vi "Execute.vi"(8 "error in (no error)":errorcluster, 10 "Notify Plugins of Menu Up in":refnum<class "Notify Plugins of Menu Up.lvclass">, 11 "Plugin Handler Shifter Data Definition":T1) -> (0 "error out":errorcluster, 1 "Stop?":bool, 2 "Plugin Generic Command out":refnum<class "Plugin Handler Command.lvclass">, 3 "Plugin Handler Shifter Data Out":T1)   [LabVIEW 2011, in "Notify Plugins of Menu Up.lvclass"]
uses:
  Notify Plugins of Menu Up.lvclass
  Plugin Handler Command.lvclass
  Plugin Strict Type Definitions/Plugin Handler Shifter Data Definition.ctl
  Parent Plugin Definition/Plugin Template/Generic Plugin.lvclass
  Plugin Strict Type Definitions/Plugin Configuration Information.ctl
  User Interface/UI Command Manager/UI Command Manager.lvclass
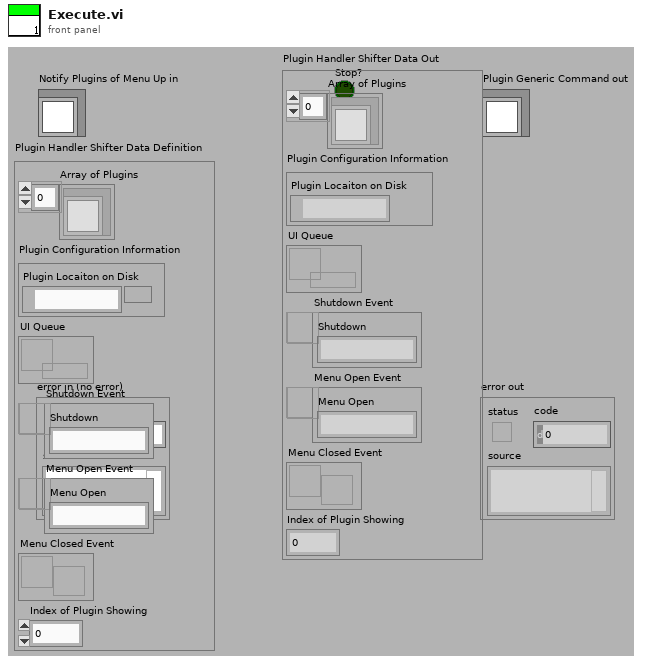
[diagram p1: front panel]
types:
  T1 = typedef "Plugin Handler Shifter Data Definition.ctl" = cluster{"Array of Plugins":refnum<class "Generic Plugin.lvclass">[], "Plugin Configuration Information":T2, "UI Queue":refnum<queue>, "Shutdown Event":refnum<user-event>, "Menu Open Event":refnum<user-event>, "Menu Closed Event":refnum<user-event>, "Index of Plugin Showing":i32}
  T2 = typedef "Plugin Configuration Information.ctl" = cluster{"Plugin Locaiton on Disk":path}
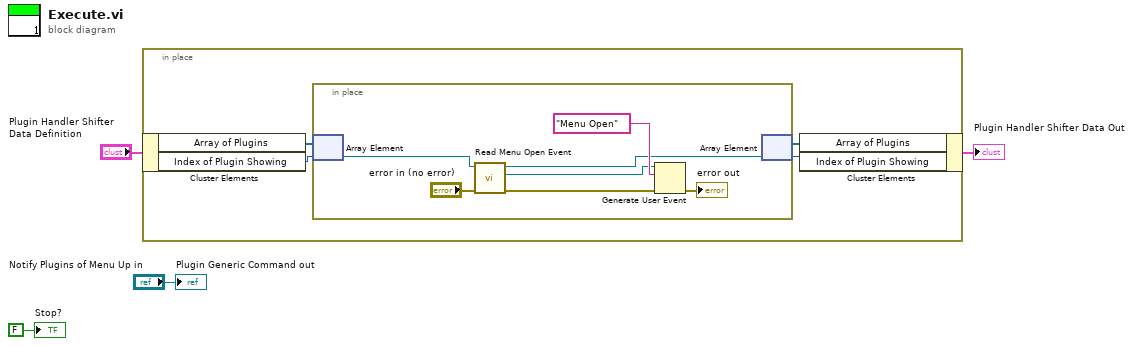
[diagram p0: block diagram]
diagram:
  n1 = in-place {
    n2 = in-place-cluster #1("Plugin Handler Shifter Data Definition") -> ("Array of Plugins"=w8:refnum<class "Generic Plugin.lvclass">[], "Index of Plugin Showing"=w7:i32)
    n3 = in-place {
      n4 = in-place-array #2(w8, w7) -> (w13:refnum<class "Generic Plugin.lvclass">)
      n5 = call "Read Menu Open Event.vi"("error in (no error)"="error in (no error)", "Generic Plugin in"=w13) -> ("error out"=w14:errorcluster, "Menu Open Event"=w12:refnum<user-event>, "Generic Plugin out"=w11:refnum<class "Generic Plugin.lvclass">)  [unwired: 7 in]
      n6 = Generate User Event(user event=w12, event data cluster="Menu Open" ("event data"), error in=w14) -> (error out=→"error out":errorcluster)  [unwired: 1 out]
      n7 = in-place-array #2(w11) -> (w6:refnum<class "Generic Plugin.lvclass">[], w5:i32)
    }
    n8 = in-place-cluster #1("Array of Plugins"=w6, "Index of Plugin Showing"=w5) -> (→"Plugin Handler Shifter Data Out":T1)
  }
  "Plugin Generic Command out" <- "Notify Plugins of Menu Up in"
  "Stop?" <- FALSE ("Stop?")
